vi "code to enum.vi"(11 "code":i32) -> (1 "valid?":bool, 2 "severity":T1, 3 "file error":T2)   [LabVIEW 2013, in "file errors.lvlib"]
uses:
  file errors.lvlib
  file error.ctl
  severity.ctl
  exception.lvlib
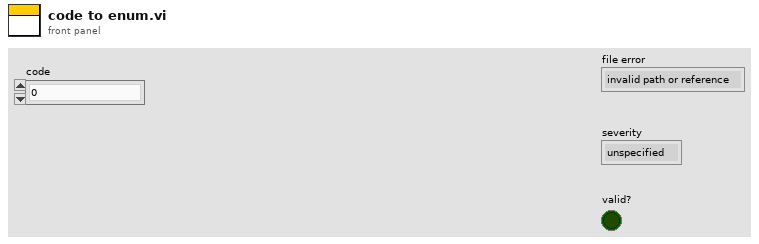
[diagram p1: front panel]
types:
  T1 = typedef "exception.lvlib/severity.ctl" = enum8{"unspecified", "informational", "operation failed", "data corruption", "system corruption", "critical unknown state"}
  T2 = typedef "file errors.lvlib/file error.ctl" = enum16{"invalid path or reference", "end of file", "file already opened", "generic file error", "file not found", "permissions invalid", "disk full", "duplicate path", "too many open file handles", "useless generic error"}
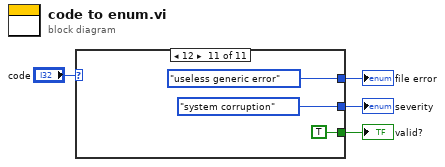
[diagram p0: block diagram]
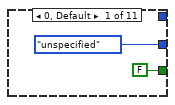
[diagram p2: hidden frame]
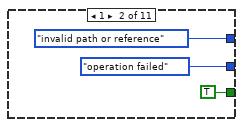
[diagram p3: hidden frame]
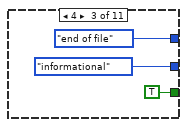
[diagram p4: hidden frame]
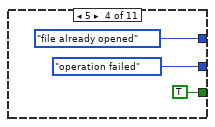
[diagram p5: hidden frame]
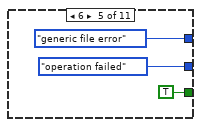
[diagram p6: hidden frame]
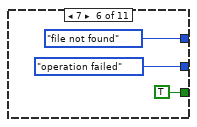
[diagram p7: hidden frame]
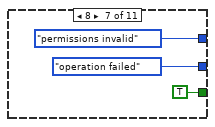
[diagram p8: hidden frame]
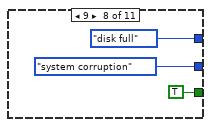
[diagram p9: hidden frame]
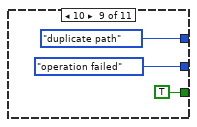
[diagram p10: hidden frame]
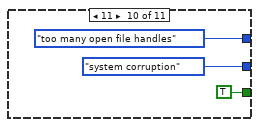
[diagram p11: hidden frame]
diagram:
  n1 = case shown="12" "code" {
    tunnel: [FALSE TRUE TRUE TRUE TRUE TRUE TRUE TRUE TRUE TRUE TRUE] -> w3
    tunnel: [_ file_error."invalid path or reference" ("file error") file_error."end of file" ("file error") file_error."file already opened" ("file error") file_error."generic file error" ("file error") file_error."file not found" ("file error") file_error."permissions invalid" ("file error") file_error."disk full" ("file error") file_error."duplicate path" ("file error") file_error."too many open file handles" ("file error") file_error."useless generic error" ("file error")] -> w2
    tunnel: [severity."unspecified" ("severity") severity."operation failed" ("severity") severity."informational" ("severity") severity."operation failed" ("severity") severity."operation failed" ("severity") severity."operation failed" ("severity") severity."operation failed" ("severity") severity."system corruption" ("severity") severity."operation failed" ("severity") severity."system corruption" ("severity") severity."system corruption" ("severity")] -> w1
    frame 0, Default {
    }
    frame 1 {
    }
    frame 4 {
    }
    frame 5 {
    }
    frame 6 {
    }
    frame 7 {
    }
    frame 8 {
    }
    frame 9 {
    }
    frame 10 {
    }
    frame 11 {
    }
    frame 12 {
    }
  }
  "file error" <- w2
  "valid?" <- w3
  "severity" <- w1
